vi "PopulateUserList.vi"(8 "error in (no error)":errorcluster, 11 "Variant":variant) -> (0 "error out":errorcluster, 3 "Array":string[](array[string]))   [LabVIEW 2013]
uses:
  Connection Handler/ctl_ClientState.ctl
  Connection Handler/Connection Handler.lvlib
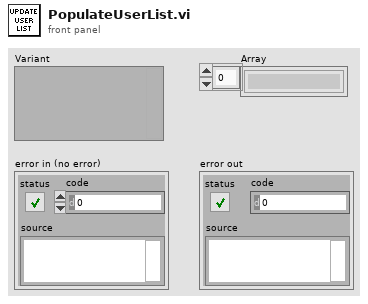
[diagram p1: front panel]
types:
  T1 = typedef "Connection Handler.lvlib/ctl_ClientState.ctl" = cluster{"Conn Ref":refnum<k5>, "IP Address":string, "Hostname":string, "User":cluster{"Username":string, "Read":bool, "Write":bool}}
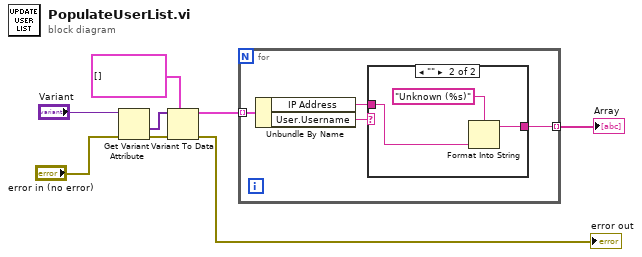
[diagram p0: block diagram]
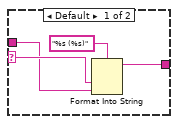
[diagram p2: hidden frame]
diagram:
  n1 = Get Variant Attribute(Variant="Variant", error in="error in (no error)") -> (values=w3:variant[], error out=w2:errorcluster)  [unwired: 2 in, 2 out]
  n2 = Variant To Data(error in=w2, type=T1[] [], Variant=w3) -> (data=w5:T1[], error out=→"error out":errorcluster)
  n3 = for {
    tunnel: w5 -> [w12] mode=indexing
    tunnel: [w10] -> w6 mode=indexing
    n4 = Unbundle By Name(w12) -> ("IP Address"=w9:string, "User.Username"=w11:string)
    n5 = case shown="\"\"" w11 {
      selector: w11 -> [w14 _]
      tunnel: [w15 w19] -> w10
      tunnel: w9 -> [w13 w17]
      frame Default {
        n6 = Format Into String(format string="%s (%s)", w14, w13) -> (resulting string=w15:string)  [unwired: 2 in, 1 out]
      }
      frame "" {
        n7 = Format Into String(format string="Unknown (%s)", w17) -> (resulting string=w19:string)  [unwired: 2 in, 1 out]
      }
    }
  }
  "Array" <- w6
